vi "Close File.vi"(8 "error in (no error)":errorcluster, 11 "Text File Sink in":refnum<class "Text File Sink.lvclass">) -> (0 "error out":errorcluster, 3 "Text File Sink out":refnum<class "Text File Sink.lvclass">)   [LabVIEW 2019, in "Text File Sink.lvclass"]
doc: "--\nCopyright © 2017 Composed SystemsI All rights reserved.\n\nAuthor: Jon McBee <jon.mcbee@composed.io>\n\nThis library is provided \"AS IS\" ,WITHOUT WARRANTIES OR\nCONDITIONS OF ANY KIND, either express or implied.\n\nComposed Systems -- composed.io\n\nStream 0.0.1.1\nJon McBee - Composed Systems\nCopyright (c) 2017, Composed Systems"
uses:
  <vilib>/gpm_packages/@cs/event-logger/Source/Text File Sink/Text File Sink.lvclass
  <vilib>/gpm_packages/@cs/event-logger/Source/Text File Sink/Text File Sink.lvclass/Text File Sink.ctl
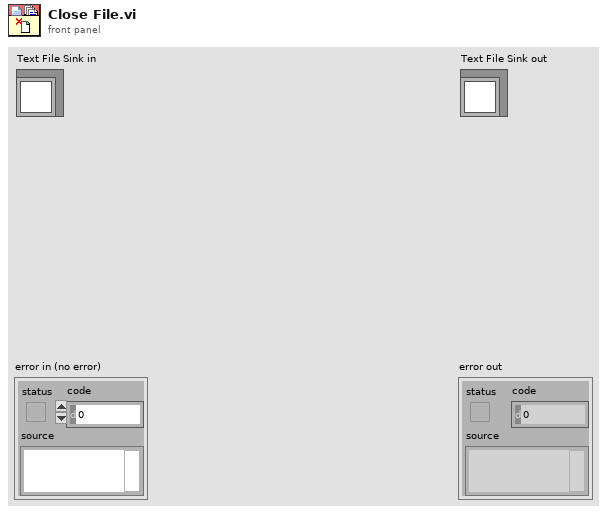
[diagram p1: front panel]
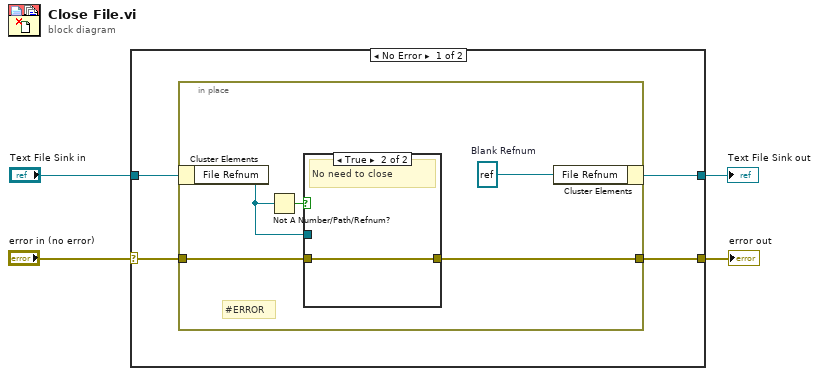
[diagram p0: block diagram]
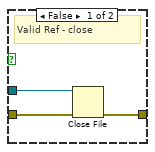
[diagram p2: hidden frame]
diagram:
  n1 = case shown="No Error" "error in (no error)" {
    selector: "error in (no error)" -> [w8 w19]
    tunnel: [w7 w19] -> w3
    tunnel: [w5 w18] -> w1
    tunnel: "Text File Sink in" -> [w6 w18]
    frame No Error {
      n2 = in-place {
        in-place-border: w8 -> [w12]
        in-place-border: [w11] -> w7
        w9 = refnum<file> refnum  # Blank Refnum
        # "#ERROR"
        n3 = in-place-cluster #1(w6) -> ("File Refnum"=w10:refnum<file>)
        n4 = Not A Number/Path/Refnum?(number/path/refnum=w10) -> (NaN/Path/Refnum?=w13:bool)
        n5 = case shown="True" w13 {
          tunnel: w12 -> [w16 w17]
          tunnel: [w15 w17] -> w11
          tunnel: w10 -> [w14 _]
          frame False {
            # "Valid Ref - close"
            n6 = Close File(refnum=w14, error in=w16) -> (error out=w15:errorcluster)  [unwired: 1 out]
          }
          frame True {
            # "No need to close"
          }
        }
        n7 = in-place-cluster #1("File Refnum"=w9) -> (w5:refnum<class "Text File Sink.lvclass">)
      }
    }
    frame Error {
    }
  }
  "error out" <- w3
  "Text File Sink out" <- w1
